vi "Stop Core.vi"(10 "final error code":i32, 11 "SignalProcessing In":refnum<class "SignalProcessing.lvclass">) -> (3 "SignalProcessing Out":refnum<class "SignalProcessing.lvclass">)   [LabVIEW 2019, in "SignalProcessing.lvlib" / "SignalProcessing.lvclass"]
doc: "(<B>Filename</B>: Actor Framework.lvlib:Actor.lvclass:Stop Core.vi)\n\nDefines what the actor does before it stops. Use the <B>final error code</B> input to determine whether the actor shut down in response to an error.\n\nBy default, this method does nothing. A descendant class may override it to define behavior, such as shutting down any processes the actor initiated in its override of the Actor Core method."
uses:
  SignalProcessing.lvclass
  SignalProcessing.lvclass/SignalProcessing.ctl
  ca78a4cf-7545-47f4-8994-d2befa69a8fd.vi
  SignalProcessing Global.vi
  <vilib>/NI/Event Source Actor/Event Source/Event Source/Event Source.lvclass
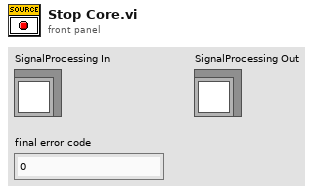
[diagram p1: front panel]
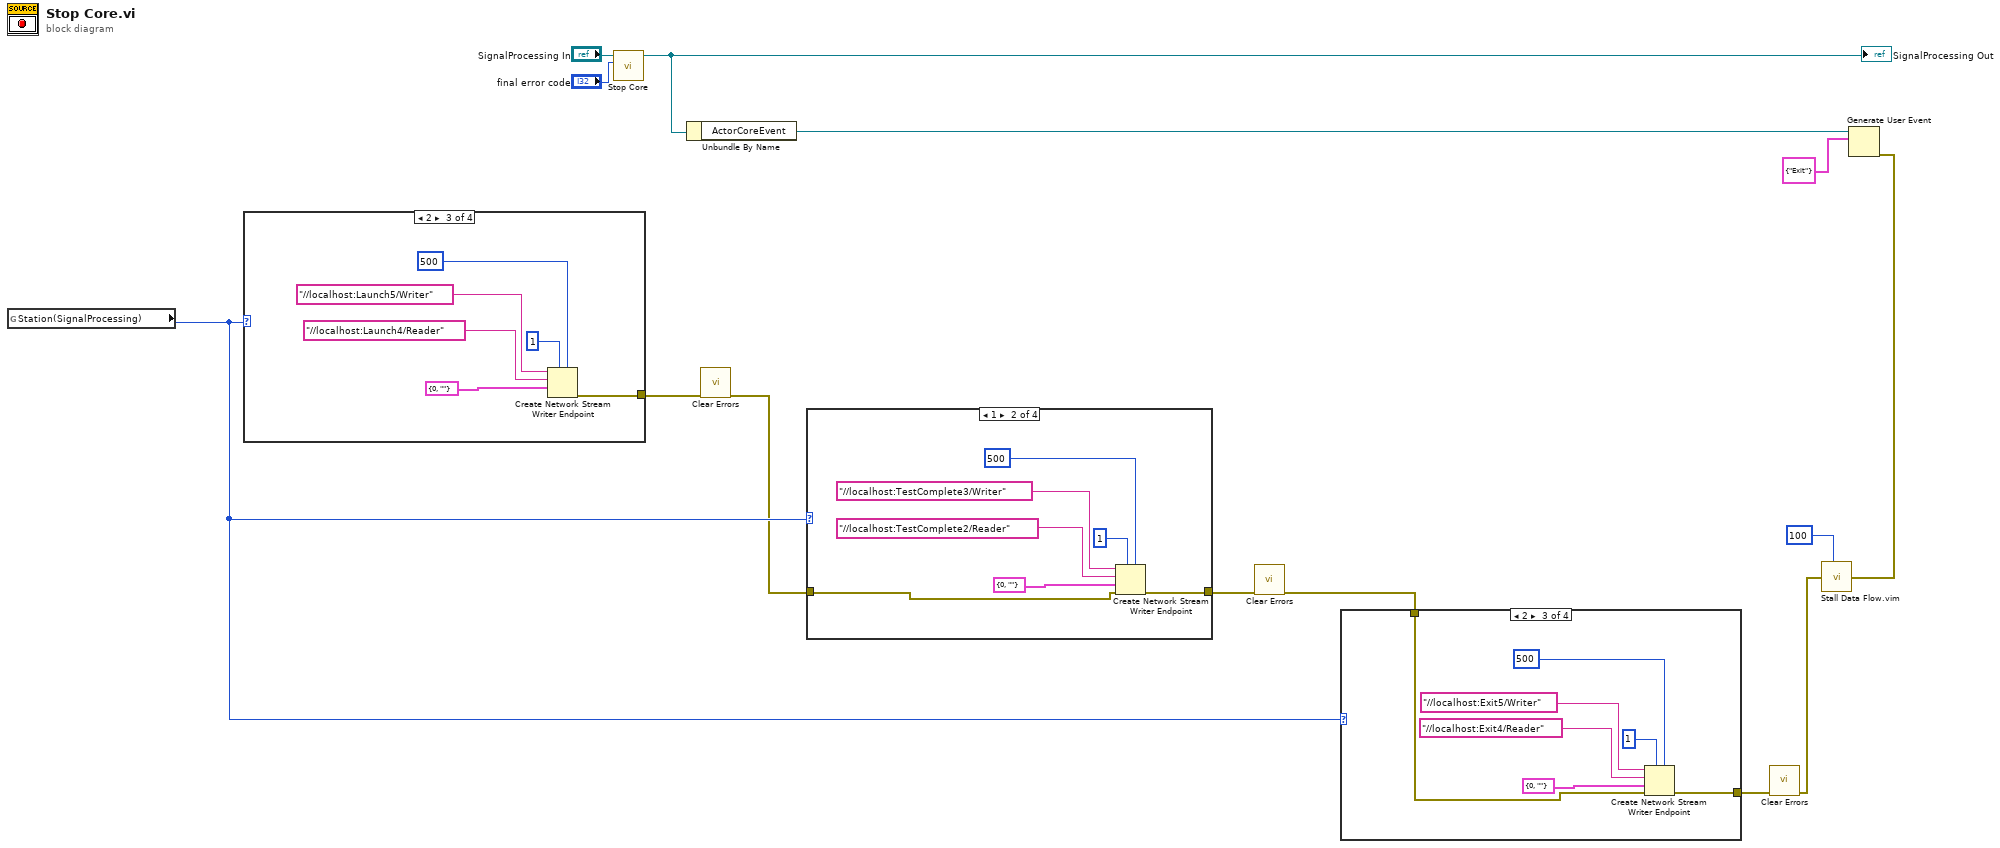
[diagram p0: block diagram]
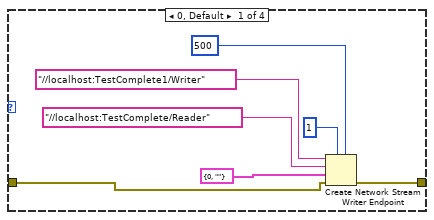
[diagram p2: hidden frame]
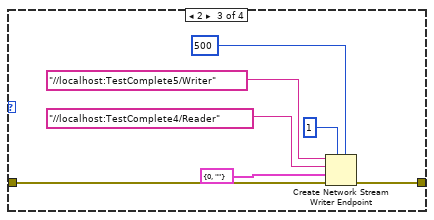
[diagram p3: hidden frame]
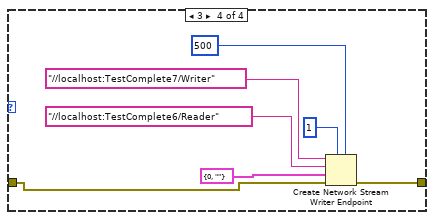
[diagram p4: hidden frame]
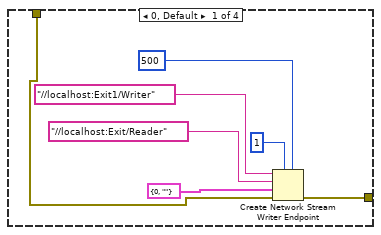
[diagram p5: hidden frame]
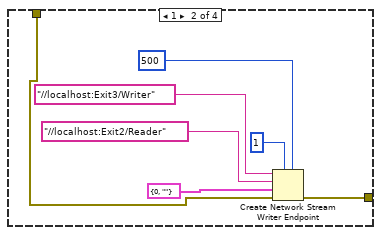
[diagram p6: hidden frame]
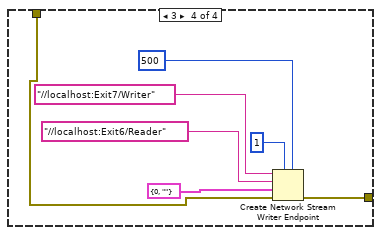
[diagram p7: hidden frame]
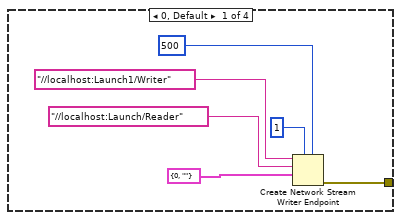
[diagram p8: hidden frame]
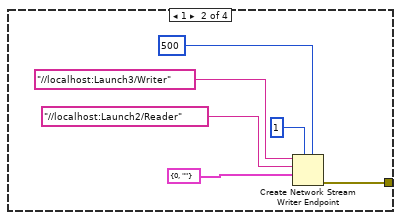
[diagram p9: hidden frame]
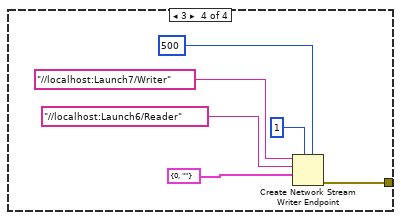
[diagram p10: hidden frame]
diagram:
  n1 = global read "SignalProcessing Global.vi" "Station(SignalProcessing)"() -> (w4:i32)
  n2 = case shown="2" w4 {
    tunnel: [w15 w21 w27 w33] -> w7
    frame 0, Default {
      n3 = Create Network Stream Writer Endpoint(5:500 ("timeout in ms (-1)"), 7:1 ("writer buffer size"), 9:cluster{"Socket":i32, "Info":string} {"Socket"=0, "Info"=""}, 10:"//localhost:Launch/Reader" ("reader name"), 11:"//localhost:Launch1/Writer" ("reader name")) -> (0:w15:errorcluster)  [unwired: 2 in, 1 out]
    }
    frame 1 {
      n4 = Create Network Stream Writer Endpoint(5:500 ("timeout in ms (-1)"), 7:1 ("writer buffer size"), 9:cluster{"Socket":i32, "Info":string} {"Socket"=0, "Info"=""}, 10:"//localhost:Launch2/Reader" ("reader name"), 11:"//localhost:Launch3/Writer" ("reader name")) -> (0:w21:errorcluster)  [unwired: 2 in, 1 out]
    }
    frame 2 {
      n5 = Create Network Stream Writer Endpoint(5:500 ("timeout in ms (-1)"), 7:1 ("writer buffer size"), 9:cluster{"Socket":i32, "Info":string} {"Socket"=0, "Info"=""}, 10:"//localhost:Launch4/Reader" ("reader name"), 11:"//localhost:Launch5/Writer" ("reader name")) -> (0:w27:errorcluster)  [unwired: 2 in, 1 out]
    }
    frame 3 {
      n6 = Create Network Stream Writer Endpoint(5:500 ("timeout in ms (-1)"), 7:1 ("writer buffer size"), 9:cluster{"Socket":i32, "Info":string} {"Socket"=0, "Info"=""}, 10:"//localhost:Launch6/Reader" ("reader name"), 11:"//localhost:Launch7/Writer" ("reader name")) -> (0:w33:errorcluster)  [unwired: 2 in, 1 out]
    }
  }
  n7 = call-parent "Stop Core.vi"("final error code"="final error code", "Event Source In"="SignalProcessing In") -> ("Event Source Out"=w12:refnum<class "SignalProcessing.lvclass">)  [unwired: 9 in]
  "SignalProcessing Out" <- w12
  n8 = Unbundle By Name(w12) -> ("ActorCoreEvent"=w11:refnum<user-event>)
  n9 = call <vilib>:"Clear Errors.vi"("error in (no error)"=w7) -> ("error out"=w3:errorcluster)  [unwired: 5 in, 1 out]
  n10 = case shown="1" w4 {
    tunnel: [w42 w49 w56 w63] -> w2
    tunnel: w3 -> [w39 w46 w55 w60]
    frame 0, Default {
      n11 = Create Network Stream Writer Endpoint(5:500 ("timeout in ms (-1)"), 7:1 ("writer buffer size"), 8:w39, 9:cluster{"Socket":i32, "Info":string} {"Socket"=0, "Info"=""}, 10:"//localhost:TestComplete/Reader" ("reader name"), 11:"//localhost:TestComplete1/Writer" ("reader name")) -> (0:w42:errorcluster)  [unwired: 1 in, 1 out]
    }
    frame 1 {
      n12 = Create Network Stream Writer Endpoint(5:500 ("timeout in ms (-1)"), 7:1 ("writer buffer size"), 8:w46, 9:cluster{"Socket":i32, "Info":string} {"Socket"=0, "Info"=""}, 10:"//localhost:TestComplete2/Reader" ("reader name"), 11:"//localhost:TestComplete3/Writer" ("reader name")) -> (0:w49:errorcluster)  [unwired: 1 in, 1 out]
    }
    frame 2 {
      n13 = Create Network Stream Writer Endpoint(5:500 ("timeout in ms (-1)"), 7:1 ("writer buffer size"), 8:w55, 9:cluster{"Socket":i32, "Info":string} {"Socket"=0, "Info"=""}, 10:"//localhost:TestComplete4/Reader" ("reader name"), 11:"//localhost:TestComplete5/Writer" ("reader name")) -> (0:w56:errorcluster)  [unwired: 1 in, 1 out]
    }
    frame 3 {
      n14 = Create Network Stream Writer Endpoint(5:500 ("timeout in ms (-1)"), 7:1 ("writer buffer size"), 8:w60, 9:cluster{"Socket":i32, "Info":string} {"Socket"=0, "Info"=""}, 10:"//localhost:TestComplete6/Reader" ("reader name"), 11:"//localhost:TestComplete7/Writer" ("reader name")) -> (0:w63:errorcluster)  [unwired: 1 in, 1 out]
    }
  }
  n15 = call <vilib>:"Clear Errors.vi"("error in (no error)"=w2) -> ("error out"=w1:errorcluster)  [unwired: 5 in, 1 out]
  n16 = case shown="2" w4 {
    tunnel: [w68 w75 w82 w89] -> w6
    tunnel: w1 -> [w67 w74 w81 w88]
    frame 0, Default {
      n17 = Create Network Stream Writer Endpoint(5:500 ("timeout in ms (-1)"), 7:1 ("writer buffer size"), 8:w67, 9:cluster{"Socket":i32, "Info":string} {"Socket"=0, "Info"=""}, 10:"//localhost:Exit/Reader" ("reader name"), 11:"//localhost:Exit1/Writer" ("reader name")) -> (0:w68:errorcluster)  [unwired: 1 in, 1 out]
    }
    frame 1 {
      n18 = Create Network Stream Writer Endpoint(5:500 ("timeout in ms (-1)"), 7:1 ("writer buffer size"), 8:w74, 9:cluster{"Socket":i32, "Info":string} {"Socket"=0, "Info"=""}, 10:"//localhost:Exit2/Reader" ("reader name"), 11:"//localhost:Exit3/Writer" ("reader name")) -> (0:w75:errorcluster)  [unwired: 1 in, 1 out]
    }
    frame 2 {
      n19 = Create Network Stream Writer Endpoint(5:500 ("timeout in ms (-1)"), 7:1 ("writer buffer size"), 8:w81, 9:cluster{"Socket":i32, "Info":string} {"Socket"=0, "Info"=""}, 10:"//localhost:Exit4/Reader" ("reader name"), 11:"//localhost:Exit5/Writer" ("reader name")) -> (0:w82:errorcluster)  [unwired: 1 in, 1 out]
    }
    frame 3 {
      n20 = Create Network Stream Writer Endpoint(5:500 ("timeout in ms (-1)"), 7:1 ("writer buffer size"), 8:w88, 9:cluster{"Socket":i32, "Info":string} {"Socket"=0, "Info"=""}, 10:"//localhost:Exit6/Reader" ("reader name"), 11:"//localhost:Exit7/Writer" ("reader name")) -> (0:w89:errorcluster)  [unwired: 1 in, 1 out]
    }
  }
  n21 = call <vilib>:"Clear Errors.vi"("error in (no error)"=w6) -> ("error out"=w5:errorcluster)  [unwired: 5 in, 1 out]
  n22 = call "Stall Data Flow.vim"("value in"=w5, "milliseconds to wait"=u32 100) -> ("value out"=w9:errorcluster)  [unwired: 1 out]
  n23 = Generate User Event(user event=w11, event data cluster=cluster{"ActorCoreMessage":string} {"ActorCoreMessage"="Exit"} ("event data"), error in=w9) -> ()  [unwired: 1 in, 2 out]
